vi "feedback loop.vi"() -> ()   [LabVIEW 2020]
panel:
  in  "Numeric 3":dbl
  out "Numeric 2":dbl
  out "Numeric":dbl
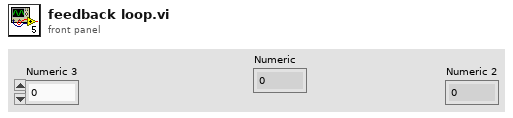
[diagram p1: front panel]
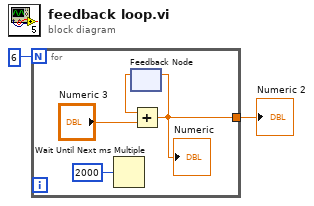
[diagram p0: block diagram]
diagram:
  n1 = for {
    N: 6 -> [_]
    tunnel: [w3] -> w1
    n2 = Wait Until Next ms Multiple(millisecond multiple=u32 2000) -> ()  [unwired: 1 out]
    n3 = feedback #1() -> (w4:dbl)  [unwired: 1 in]
    n4 = Add(x=w4, y="Numeric 3") -> (x+y=w3:dbl)
    "Numeric" <- w3
    n5 = feedback-in #1(w3) -> ()
  }
  "Numeric 2" <- w1
